vi "Spinner.vi"() -> (3 "element":string)   [LabVIEW 2019]
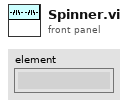
[diagram p1: front panel]
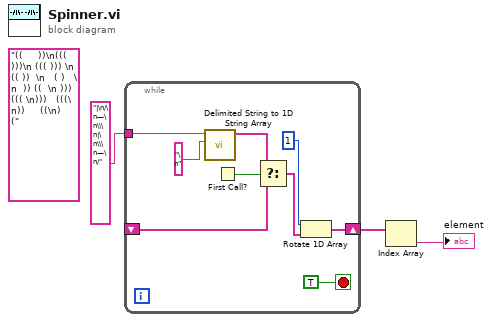
[diagram p0: block diagram]
diagram:
  (unwired) "((     ))\n(((   )))\n ((( ))) \n  (( ))  \n   ( )   \n  )) ((  \n ))) ((( \n)))   (((\n))     ((\n)       (" ("format string")
  n1 = while {
    shift-right: [w10] -> w3
    shift-left: _ -> [w7]
    tunnel: "|\n/\n—\n\\\n|\n\\\n—\n/" ("format string") -> [w4]
    stop <- TRUE stop-if-true
    n2 = call <vilib>:"Delimited String to 1D String Array.vi"("delimiter"="\n", "delimited string"=w4) -> ("string array"=w8:string[])  [unwired: 9 in]
    n3 = First Call?() -> (First Call?: T/F=w9:bool)
    n4 = Select(t=w8, s=w9, f=w7) -> (s? t:f=w6:string[])
    n5 = Rotate 1D Array(1:w6, 2:1 ("n")) -> (0:w10:string[])
  }
  n6 = Index Array(array=w3) -> (element=→"element":string)  [unwired: 1 in]
